vi "Keypad Auto Pressed(LV2015).vi"(7 "Delay Time(ms)":u32=50, 8 "error in (no error)":errorcluster, 11 "Key List":u8[](array[ring]) items=["None"=0, "Backspace"=8, "Tab"=9, "Clear"=12, "Enter"=13, "Shift"=16, "Ctrl"=17, "Alt"=18, "Pause"=19, "CapsLock"=20, "Esc"=27, "Space Bar"=32, "Page Up"=33, "Page Down"=34, "End"=35, "Home"=36, "Left Arrow"=37, "Up Arrow"=38, "Right Arrow"=39, "Down Arrow"=40, "Select"=41, "Execute"=42, "Print Screen"=44, "Ins"=45, "Del"=46, "Help"=47, "0"=48, "1"=49, "2"=50, "3"=51, "4"=52, "5"=53, "6"=54, "7"=55, "8"=56, "9"=57, "A"=65, "B"=66, "C"=67, "D"=68, "E"=69, "F"=70, "G"=71, "H"=72, "I"=73, "J"=74, "K"=75, "L"=76, "M"=77, "N"=78, "O"=79, "P"=80, "Q"=81, "R"=82, "S"=83, "T"=84, "U"=85, "V"=86, "W"=87, "X"=88, "Y"=89, "Z"=90, "Left WIN"=91, "Right WIN"=92, "Right Ctrl"=93, "Sleep Key"=95, "NumKey 0"=96, "NumKey 1"=97, "NumKey 2"=98, "NumKey 3"=99, "NumKey 4"=100, "NumKey 5"=101, "NumKey 6"=102, "NumKey 7"=103, "NumKey 8"=104, "NumKey 9"=105, "NumKey *"=106, "NumKey +"=107, "NumKey Enter"=108, "NumKey -"=109, "NumKey ."=110, "NumKey /"=111, "F1"=112, "F2"=113, "F3"=114, "F4"=115, "F5"=116, "F6"=117, "F7"=118, "F8"=119, "F9"=120, "F10"=121, "F11"=122, "F12"=123, "F13"=124, "F14"=125, "F15"=126, "F16"=127, "F17"=128, "F18"=129, "F19"=130, "F20"=131, "F21"=132, "F22"=133, "F23"=134, "F24"=135, "Num Lock"=144, "Scroll Lock"=145, "Left SHIFT"=160, "Right SHIFT"=161, "Left CONTROL"=162, "Right CONTROL"=163, "Left MENU"=164, "Right MENU"=165, "Browser Back"=166, "Browser Forward"=167, "Browser Refresh"=168, "Browser Stop"=169, "Browser Search"=170, "Brower Favorites"=171, "Brower Start and Home"=172, "Volume Mute"=173, "Volume Down"=174, "Volume Up"=175, "Next Track"=176, "Previous Track"=177, "Stop Media"=178, "Play/Pause Media"=179, "Start Mail"=180, "Select Media"=181, ":;"=186, "+="=187, "<,"=188, "_-"=189, ">."=190, "?/"=191, "~`"=192, "{["=219, "|\\"=220, "}]"=221, "\"'"=222, "Attn"=246, "CrSel"=247, "ExSel"=248, "Erase EOF"=249, "Play"=250, "Zoom"=251, "PA1"=253, "Clear"=254]) -> (0 "error out":errorcluster)   [LabVIEW 2015]
uses:
  user32.dll
panel:
  # "Keypad Auto Pressed"
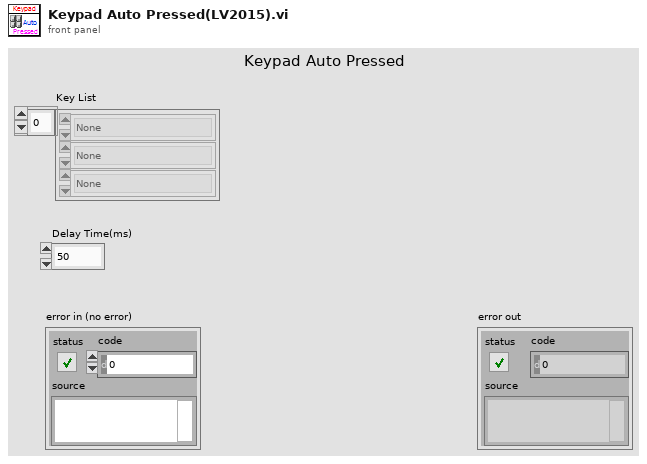
[diagram p1: front panel]
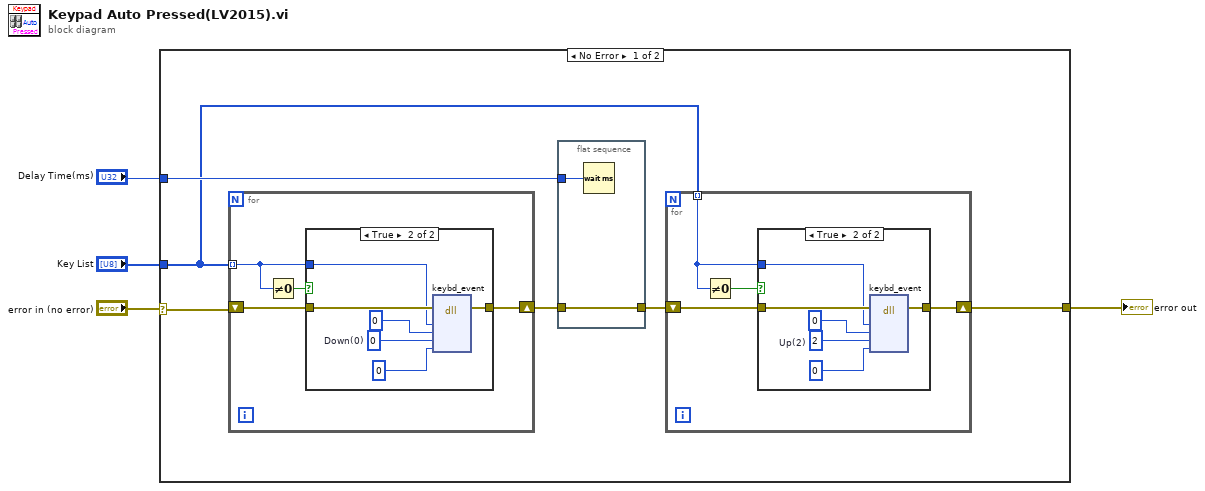
[diagram p0: block diagram]
diagram:
  n1 = case shown="No Error" "error in (no error)" {
    selector: "error in (no error)" -> [w5 w35]
    tunnel: "Delay Time(ms)" -> [w9 _]
    tunnel: "Key List" -> [w7 _]
    tunnel: [w6 w35] -> w2
    frame No Error {
      n2 = for {
        tunnel: w7 -> [w23] mode=indexing
        shift-right: [w25] -> w10
        shift-left: w5 -> [w24]
        n3 = Not Equal To 0?(x=w23) -> (x != 0?=w22:bool)
        n4 = case shown="True" w22 {
          tunnel: w24 -> [w26 w30]
          tunnel: [w26 w29] -> w25
          tunnel: w23 -> [_ w27]
          frame False {
          }
          frame True {
            w28 = u32 0  # Down(0)
            n5 = dll-call lib="user32.dll" fn="keybd_event"(error in=w30, "KeypadValue"=w27, "bScan"=u8 0, "dwflag"=w28, "swExinfo"=u32 0) -> (error out=w29:errorcluster)  [unwired: 7 in, 1 out]
          }
        }
      }
      n6 = flat-sequence {
        tunnel: [w34] -> w8
        tunnel: w10 -> [w34]
        tunnel: w9 -> [w33]
        frame #0 {
          n7 = Wait (ms)(milliseconds to wait=w33) -> ()  [unwired: 1 out]
        }
      }
      n8 = for {
        shift-right: [w14] -> w6
        shift-left: w8 -> [w13]
        tunnel: w7 -> [w11] mode=indexing
        n9 = Not Equal To 0?(x=w11) -> (x != 0?=w12:bool)
        n10 = case shown="True" w12 {
          tunnel: w13 -> [w15 w19]
          tunnel: [w15 w18] -> w14
          tunnel: w11 -> [_ w16]
          frame False {
          }
          frame True {
            w17 = u32 2  # Up(2)
            n11 = dll-call lib="user32.dll" fn="keybd_event"(error in=w19, "KeypadValue"=w16, "bScan"=u8 0, "dwflag"=w17, "swExinfo"=u32 0) -> (error out=w18:errorcluster)  [unwired: 7 in, 1 out]
          }
        }
      }
    }
    frame Error {
    }
  }
  "error out" <- w2
